vi "Initialize IO.vi"(8 "error in (no error)":errorcluster, 11 "DigitalIO in":refnum<class "DigitalIO.lvclass">) -> (0 "error out":errorcluster, 3 "DigitalIO out":refnum<class "DigitalIO.lvclass">)   [LabVIEW 2018, in "DigitalIO.lvlib" / "DigitalIO.lvclass"]
uses:
  DigitalIO.lvclass
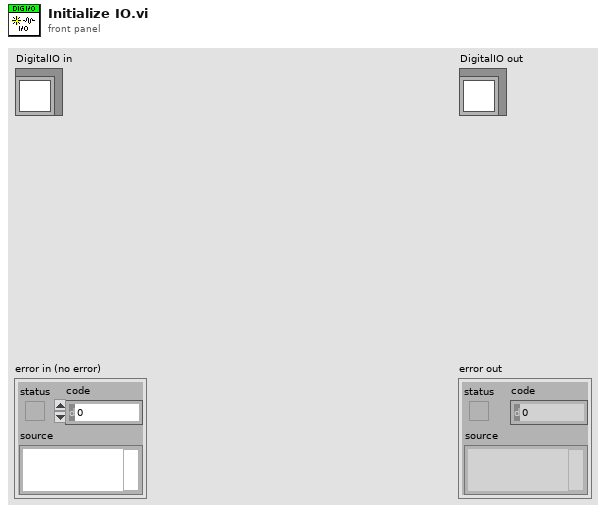
[diagram p1: front panel]
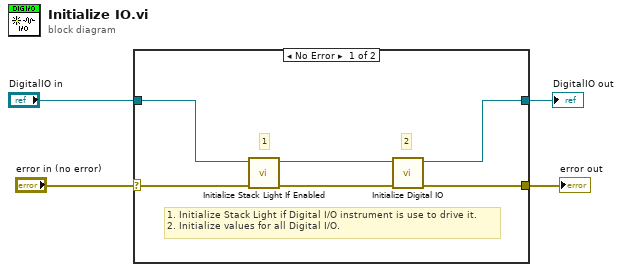
[diagram p0: block diagram]
diagram:
  n1 = case shown="No Error" "error in (no error)" {
    selector: "error in (no error)" -> [w10 w12]
    tunnel: [w6 w12] -> w3
    tunnel: [w5 w11] -> w1
    tunnel: "DigitalIO in" -> [w9 w11]
    frame No Error {
      # "1. Initialize Stack Light if Digital I/O instrument is use to drive it.\n2. Initialize values for all Digital I/O."
      # "2"
      # "1"
      n2 = call "Initialize Stack Light If Enabled.vi"("error in (no error)"=w10, "DigitalIO in"=w9) -> ("error out"=w8:errorcluster, "DigitalIO out"=w7:refnum<class "DigitalIO.lvclass">)  [unwired: 8 in]
      n3 = call "Initialize Digital IO.vi"("error in (no error)"=w8, "DigitalIO in"=w7) -> ("error out"=w6:errorcluster, "DigitalIO out"=w5:refnum<class "DigitalIO.lvclass">)  [unwired: 8 in]
    }
    frame Error {
    }
  }
  "error out" <- w3
  "DigitalIO out" <- w1
